vi "Coerced with Sign.vi"(0 "Input":dbl format="%#_13g", 3 "Limits":cluster{"\"Upper\"":dbl, "\"Lower\"":dbl}={"\"Upper\""=0.7, "\"Lower\""=0.05}) -> (7 "Coerced":dbl format="%#_13g", 10 "In Range?":bool)   [LabVIEW 2015]
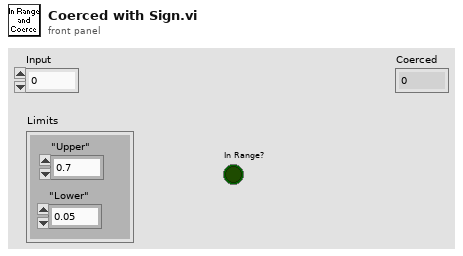
[diagram p1: front panel]
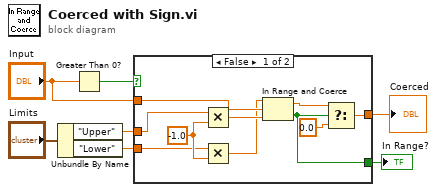
[diagram p0: block diagram]
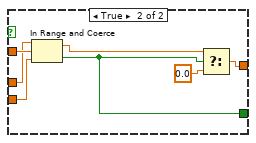
[diagram p2: hidden frame]
diagram:
  n1 = Unbundle By Name("Limits") -> ("\"Upper\""=w5:dbl, "\"Lower\""=w4:dbl)
  n2 = Greater Than 0?(x="Input") -> (x > 0?=w6:bool)
  n3 = case shown="False" w6 {
    tunnel: w5 -> [w17 w20]
    tunnel: w4 -> [w15 w19]
    tunnel: [w12 w22] -> w3
    tunnel: "Input" -> [w14 w24]
    tunnel: [w8 w18] -> w1
    frame False {
      w16 = -1.0
      n4 = Multiply(x=w17, y=w16) -> (x*y=w10:dbl)
      n5 = Multiply(x=w15, y=w16) -> (x*y=w9:dbl)
      n6 = In Range and Coerce(upper limit=w9, x=w14, lower limit=w10) -> (coerced(x)=w13:dbl, In Range?=w8:bool)
      n7 = Select(t=w13, s=w8, f=0.0) -> (s? t:f=w12:dbl)
    }
    frame True {
      n8 = In Range and Coerce(upper limit=w20, x=w24, lower limit=w19) -> (coerced(x)=w21:dbl, In Range?=w18:bool)
      n9 = Select(t=w21, s=w18, f=0.0) -> (s? t:f=w22:dbl)
    }
  }
  "Coerced" <- w3
  "In Range?" <- w1
